vi "WriteAllStepSetupClusterArray.vi"(8 "error in (no error)":errorcluster, 10 "AllStepSetupClusterArray":T1 {"AllStepTypeData"."MoveData"."Mode" items=["Abs"=2, "Inc"=3]; "AllStepTypeData"."MoveData"."Axis" items=["X"=1, "Y"=2, "Z"=3, "Rotation"=4]}, 11 "StepData.lvclass In":refnum<class "StepData.lvclass">) -> (0 "error out":errorcluster, 3 "StepData.lvclass Out":refnum<class "StepData.lvclass">)   [LabVIEW 2014, in "StepData.lvclass"]
uses:
  StepData.lvclass
  Project/StepSetupDataTypeDefine.ctl
  Control/AllStepTypeData.ctl
  Control/StepTypeEnum.ctl
  Control/MoveData.ctl
  Control/MeasureData.ctl
  StepData.lvclass/StepData.ctl
  Project/Project.lvclass
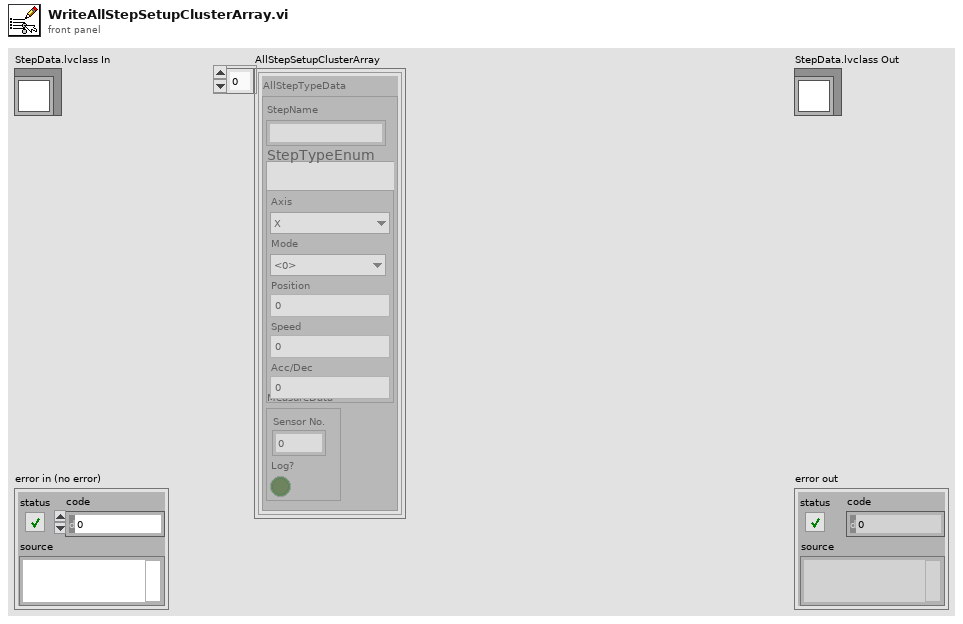
[diagram p1: front panel]
types:
  T1 = typedef "Project.lvclass/StepSetupDataTypeDefine.ctl" = cluster{"AllStepTypeData":T2}[]
  T2 = typedef "StepData.lvclass/AllStepTypeData.ctl" = cluster{"StepName":string, "StepTypeEnum":T3, "MoveData":T4, "MeasureData":T5}
  T3 = typedef "StepData.lvclass/StepTypeEnum.ctl" = enum16{"Move", "Measure"}
  T4 = typedef "StepData.lvclass/MoveData.ctl" = cluster{"Axis":u16, "Position":dbl, "Speed":dbl, "Acc/Dec":dbl, "Mode":u16}
  T5 = typedef "StepData.lvclass/MeasureData.ctl" = cluster{"Sensor No.":i32, "Log?":bool}
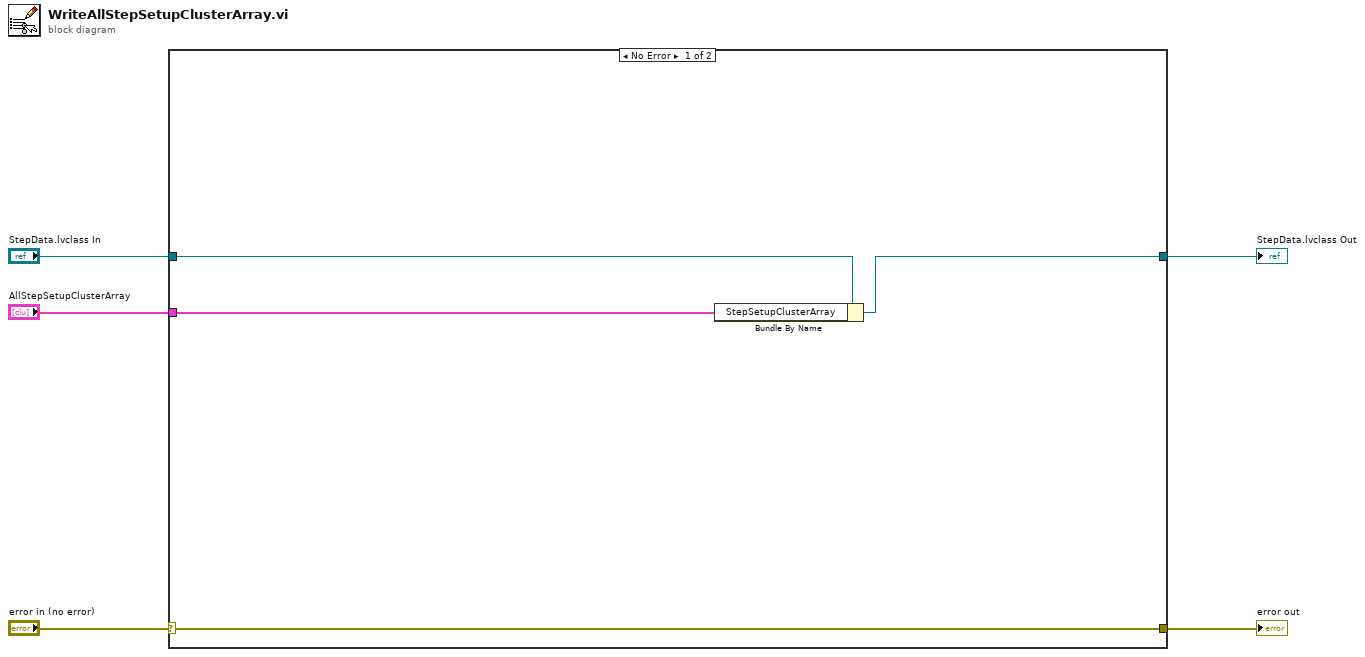
[diagram p0: block diagram]
diagram:
  n1 = case shown="No Error" "error in (no error)" {
    selector: "error in (no error)" -> [w9 w11]
    tunnel: [w9 w11] -> w4
    tunnel: "StepData.lvclass In" -> [w8 w10]
    tunnel: [w7 w10] -> w2
    tunnel: "AllStepSetupClusterArray" -> [w6 _]
    frame No Error {
      n2 = Bundle By Name(cluster=w8, "StepSetupClusterArray"=w6) -> (w7:refnum<class "StepData.lvclass">)
    }
    frame Error {
    }
  }
  "error out" <- w4
  "StepData.lvclass Out" <- w2
